vi "FlatToRichmeasurement_ProcessResponse.vi"(5 "OutputClusterType":T1, 11 "InputCluster":T2) -> (3 "OutputCluster":T1)   [LabVIEW 2021, in "Measurement_server.lvlib"]
uses:
  Measurement_server.lvlib
  measurement_ProcessResponse_Flat.ctl
  measurement_ProcessResponse.ctl
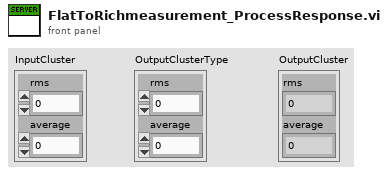
[diagram p1: front panel]
types:
  T1 = typedef "Measurement_server.lvlib/measurement_ProcessResponse.ctl" = cluster{"rms":dbl, "average":dbl}
  T2 = typedef "Measurement_server.lvlib/measurement_ProcessResponse_Flat.ctl" = cluster{"rms":dbl, "average":dbl}
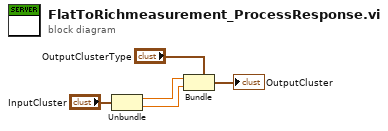
[diagram p0: block diagram]
diagram:
  n1 = Unbundle "Unbundle"("InputCluster") -> ("rms"=w2:dbl, "average"=w1:dbl)
  n2 = Bundle "Bundle"(cluster="OutputClusterType", "rms"=w2, "average"=w1) -> (→"OutputCluster":T1)
